vi "Period.set.vi"(8 "error in (no error)":errorcluster, 10 "period (ms)":i32, 11 "EventDaemon in":refnum<class "MemoryManager.lvclass">) -> (0 "error out":errorcluster, 3 "EventDaemon out":refnum<class "MemoryManager.lvclass">)   [LabVIEW 2024, in "MemoryManager.lvclass"]
doc: "Set the daemon loop period in milliseconds"
uses:
  MemoryManager.lvclass
  MemoryManager.lvclass/MemoryManager.ctl
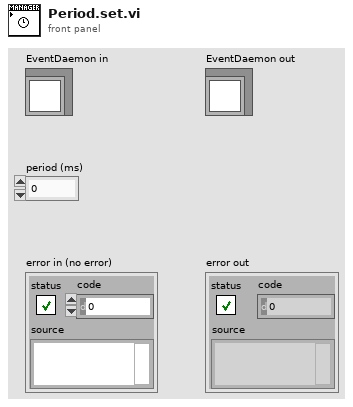
[diagram p1: front panel]
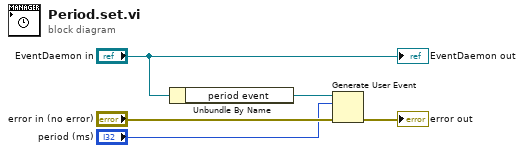
[diagram p0: block diagram]
diagram:
  n1 = Unbundle By Name("EventDaemon in") -> ("period event"=w4:refnum<user-event>)
  n2 = Generate User Event(user event=w4, event data cluster="period (ms)", error in="error in (no error)") -> (error out=→"error out":errorcluster)  [unwired: 1 in, 1 out]
  "EventDaemon out" <- "EventDaemon in"
